vi "NR_Precode.vi"(0 "appended path":path, 1 "DMRS_symbol":dbl, 3 "mod_data":cdb[](array[numeric]), 4 "CodebookTransform_en":dbl, 5 "vnum":dbl, 6 "TPMIindex":dbl, 9 "Nsym_slot":dbl, 11 "TransformPrcode_en":dbl, 12 "Antportnum":dbl, 13 "error in (no error)":errorcluster caption="错误输入（无错误）", 14 "prb_num":dbl) -> (10 "precodedata":cdb[](array[numeric]), 15 "error IO":errorcluster)   [LabVIEW 2015]
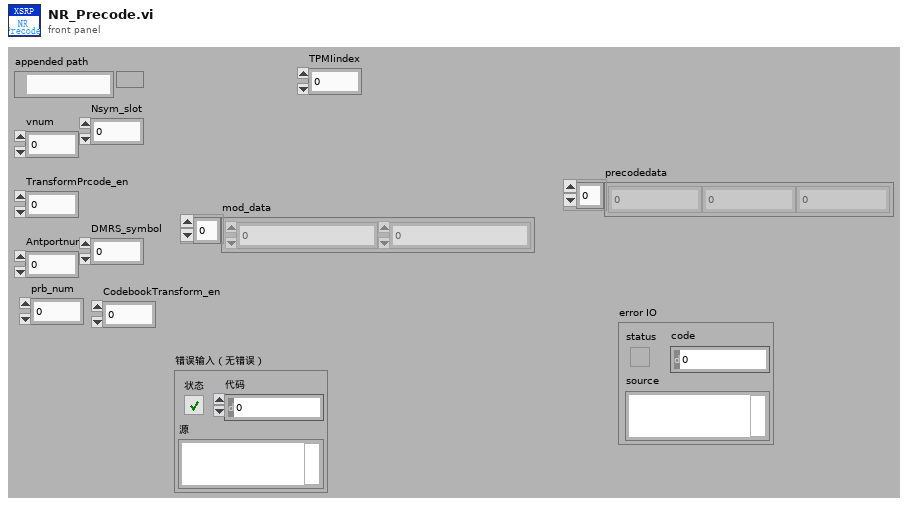
[diagram p1: front panel]
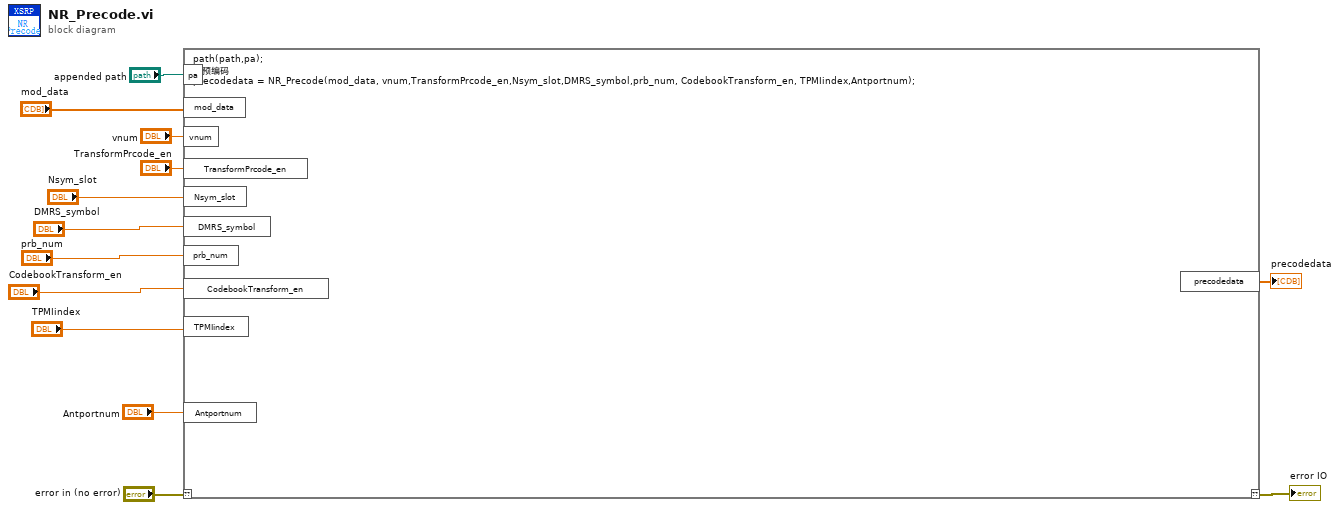
[diagram p0: block diagram]
diagram:
  n1 = script code="path(path,pa);\n%预编码\nprecodedata = NR_Precode(mod_data, vnum,TransformPrcode_en,Nsym_slot,DMRS_symbol,prb_num, CodebookTransform_en, TPMIindex,Antportnum);"("??"="error in (no error)", "pa"="appended path", "vnum"="vnum", "TransformPrcode_en"="TransformPrcode_en", "Antportnum"="Antportnum", "mod_data"="mod_data", "Nsym_slot"="Nsym_slot", "DMRS_symbol"="DMRS_symbol", "prb_num"="prb_num", "CodebookTransform_en"="CodebookTransform_en", "TPMIindex"="TPMIindex") -> ("??"=→"error IO":errorcluster, "precodedata"=→"precodedata":cdb[])
